vi "FP_Repair_broken_TDMS.vi"(8 "Error in":errorcluster caption="Error In", 11 "TDMS file to repair":path) -> (0 "Error Out":errorcluster caption="Error Out (if any)", 2 "Outcome":string caption="Outcome:")   [LabVIEW 2018]
uses:
  <vilib>/Utility/miscctls.llb/LVPointTypeDef.ctl
  <userlib>/_OpenG.lib/file/file.llb/File Exists - Scalar__ogtk.vi
  <userlib>/_OpenG.lib/file/file.llb/Valid Path - Traditional__ogtk.vi
  <userlib>/_OpenG.lib/file/file.llb/Convert File Extension (Path)__ogtk.vi
panel:
  in  "Repair":bool
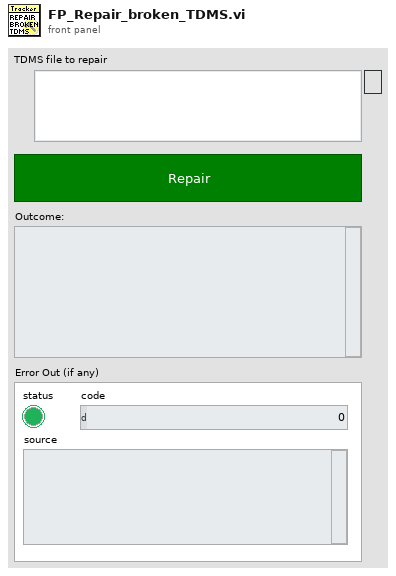
[diagram p1: front panel]
types:
  T1 = enum8{"Enabled", "Disabled", "Disabled and Grayed Out"}
  T2 = typedef "LVPointTypeDef.ctl" = cluster{"Horizontal":i16, "Vertical":i16}
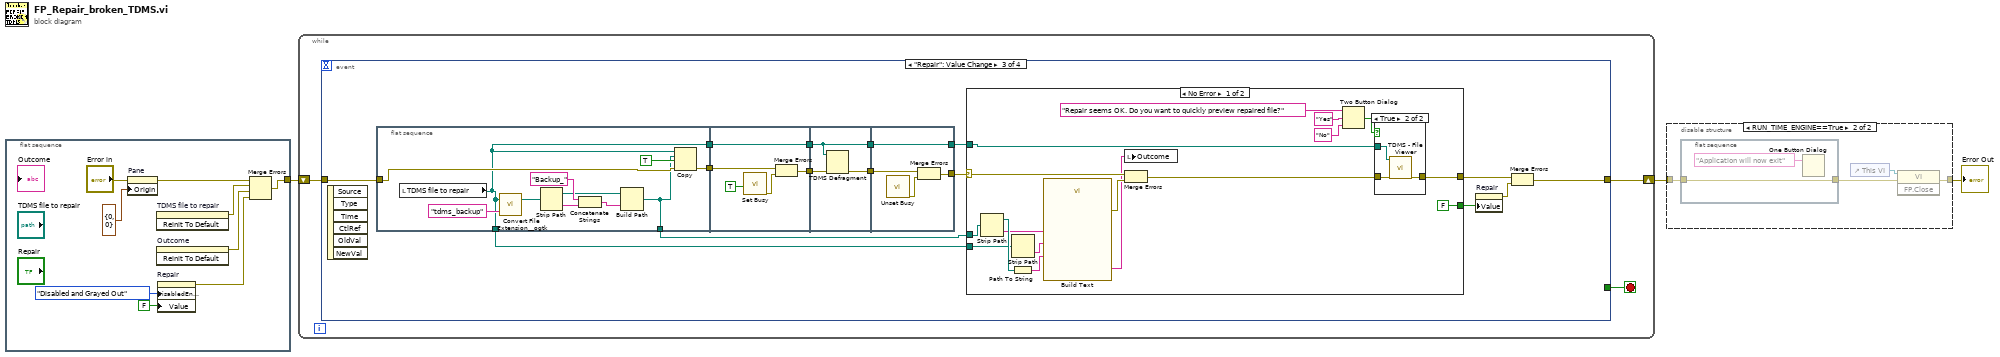
[diagram p0: block diagram]
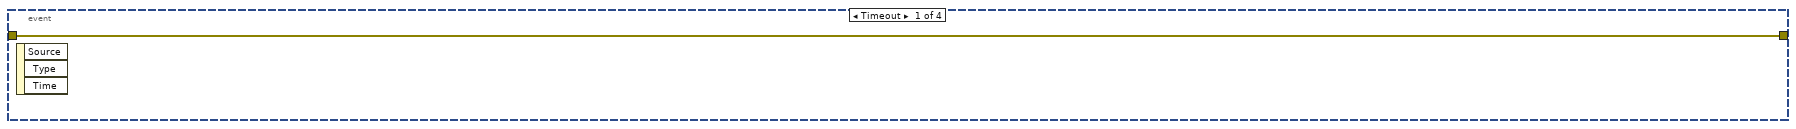
[diagram p3: hidden frame]
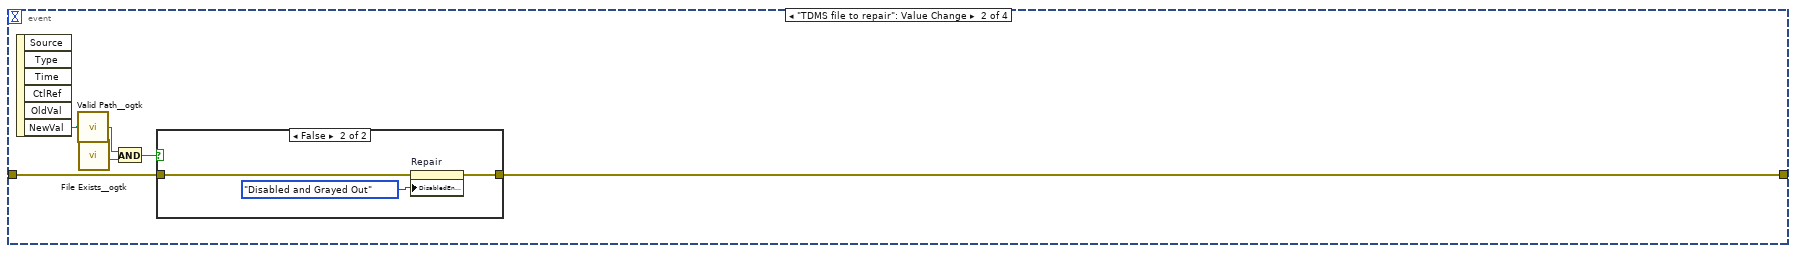
[diagram p4: hidden frame]
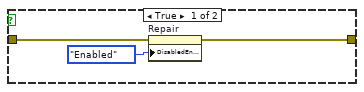
[diagram p5: hidden frame]
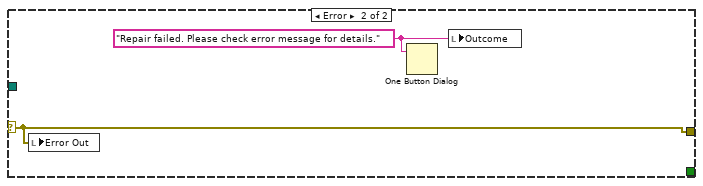
[diagram p7: hidden frame]
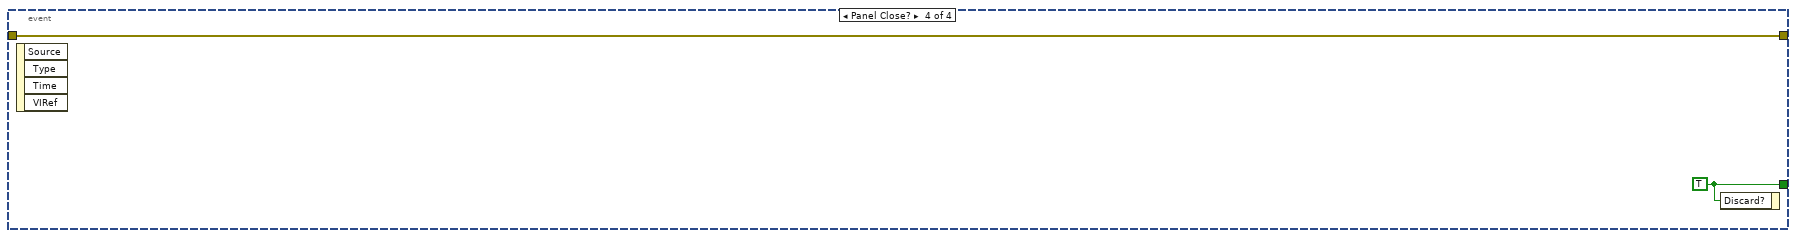
[diagram p8: hidden frame]
diagram:
  n1 = flat-sequence {
    tunnel: [w9] -> w1
    frame #0 {
      n2 = property on="Pane" class="Pane"(error in="Error in", "Origin"=T2 {"Horizontal"=0, "Vertical"=0}) -> (error out=w10:errorcluster)  [unwired: 1 in, 1 out]
      n3 = invoke on="TDMS file to repair" class="Path" method="Reinit To Default"() -> (error out=w6:errorcluster)  [unwired: 3 in, 2 out]
      n4 = invoke on="Outcome" class="Str" method="Reinit To Default"() -> (error out=w5:errorcluster)  [unwired: 3 in, 2 out]
      n5 = property on="Repair" class="Bool (strict)"("DisabledEnum"=T1."Disabled and Grayed Out" ("Disabled"), "Value"=FALSE ("Repair")) -> (error out=w4:errorcluster)  [unwired: 2 in, 1 out]
      n6 = Merge Errors(w10, w6, w5, w4) -> (w9:errorcluster)
    }
  }
  n7 = while {
    shift-right: [w14] -> w3
    shift-left: w1 -> [w13]
    stop <- w15 stop-if-true
    n8 = event shown="[2] \"Repair\": Value Change" {
      selector: _ -> [_ _ _ _]
      dyn-events: _ -> [_ _ _ _]
      timeout: _ -> [_ _ _ _]
      tunnel: [_ _ _ w91] -> w15
      tunnel: [w16 w20 w38 w90] -> w14
      tunnel: w13 -> [w16 w21 w43 w90]
      event Timeout {
        n9 = event-data() -> ()  [unwired: 1 in, 3 out]
      }
      event "TDMS file to repair": Value Change {
        n10 = event-data() -> ("NewVal"=w19:path)  [unwired: 1 in, 5 out]
        n11 = call-poly <userlib>:"Valid Path__ogtk.vi"("path"=w19) -> ("valid"=w22:bool)
        n12 = call-poly <userlib>:"File Exists__ogtk.vi"("file path"=w19) -> ("exists"=w17:bool)  [unwired: 6 in, 1 out]
        n13 = And(x=w22, y=w17) -> (x .and. y?=w18:bool)
        n14 = case shown="False" w18 {
          tunnel: w21 -> [w25 w28]
          tunnel: [w23 w26] -> w20
          frame True {
            n15 = property on="Repair" class="Bool (strict)"(error in=w25, "DisabledEnum"=T1."Enabled" ("Disabled")) -> (error out=w23:errorcluster)  [unwired: 1 in, 1 out]
          }
          frame False {
            n16 = property on="Repair" class="Bool (strict)"(error in=w28, "DisabledEnum"=T1."Disabled and Grayed Out" ("Disabled")) -> (error out=w26:errorcluster)  [unwired: 1 in, 1 out]
          }
        }
      }
      event "Repair": Value Change {
        n17 = event-data() -> ()  [unwired: 1 in, 6 out]
        n18 = flat-sequence {
          tunnel: w43 -> [w75]
          tunnel: [w74] -> w34
          tunnel: [w73] -> w32
          tunnel: [w73] -> w39
          tunnel: [w67] -> w35
          tunnel: w34 -> [w82]
          tunnel: [w79] -> w33
          tunnel: w32 -> [w81]
          tunnel: [w81] -> w31
          tunnel: w33 -> [w85]
          tunnel: w31 -> [w83]
          tunnel: [w84] -> w30
          tunnel: [w83] -> w29
          tunnel: [w88] -> w41
          tunnel: [w87] -> w42
          tunnel: w30 -> [w89]
          tunnel: w29 -> [w88]
          frame #0 {
            n19 = local read "TDMS file to repair"() -> (w73:path)
            n20 = call-poly <userlib>:"Convert File Extension__ogtk.vi"("new ending (none)"="tdms_backup", "file name"=w73) -> ("new filename"=w72:path)  [unwired: 1 out]
            n21 = Strip Path(path=w72) -> (stripped path=w68:path, name=w71:string)
            n22 = Concatenate Strings("Backup_" ("string"), w71) -> (w69:string)
            n23 = Build Path(base path=w68, name or relative path=w69) -> (appended path=w67:path)
            n24 = Copy(8:w75, 9:TRUE ("overwrite (F)"), 10:w67, 11:w73) -> (0:w74:errorcluster)  [unwired: 1 in, 2 out]
          }
          frame #1 {
            n25 = call <vilib>:"Set Busy.vi"("disable click? (T)"=TRUE) -> ("error out"=w78:errorcluster)  [unwired: 9 in, 1 out]
            n26 = Merge Errors(w82, w78) -> (w79:errorcluster)
          }
          frame #2 {
            n27 = TDMS Defragment(4:w85, 7:w83) -> (0:w84:errorcluster)
          }
          frame #3 {
            n28 = call <vilib>:"Unset Busy.vi"() -> ("error out"=w86:errorcluster)  [unwired: 11 in]
            n29 = Merge Errors(w89, w86) -> (w87:errorcluster)
          }
        }
        n30 = case shown="No Error" w42 {
          selector: w42 -> [w56 w66]
          tunnel: w41 -> [w52 _]
          tunnel: [w55 w66] -> w40
          tunnel: w39 -> [w48 _]
          tunnel: [FALSE _] -> w36
          tunnel: w35 -> [w44 _]
          frame No Error {
            n31 = Strip Path(path=w44) -> (stripped path=w51:path, name=w49:string)
            n32 = Path To String(path=w51) -> (string=w50:string)
            n33 = Strip Path(path=w48) -> (name=w47:string)  [unwired: 1 out]
            n34 = call "Build Text"("original_file"=w49, "repaired_file"=w47, "folder"=w50) -> ("Result"=w46:string, "error out"=w53:errorcluster)  [unwired: 11 in]
            n35 = local write "Outcome"(w46) -> ()
            n36 = Merge Errors(w56, w53) -> (w54:errorcluster)
            n37 = Two Button Dialog(message="Repair seems OK. Do you want to quickly preview repaired file?", 1:"No" ("F button name (\"Cancel\")"), 2:"Yes" ("T button name (\"OK\")")) -> (T button?=w59:bool)
            n38 = case shown="True" w59 {
              tunnel: w52 -> [_ w64]
              tunnel: w54 -> [w61 w63]
              tunnel: [w61 w62] -> w55
              frame False {
              }
              frame True {
                n39 = call <vilib>:"TDMS - File Viewer.vi"("error in (no error)"=w63, "file path"=w64) -> ("error out"=w62:errorcluster)  [unwired: 4 in, 1 out]
              }
            }
          }
          frame Error {
            w65 = "Repair failed. Please check error message for details." ("message")
            n40 = local write "Error Out"(w66) -> ()
            n41 = One Button Dialog(message=w65) -> ()  [unwired: 1 in, 1 out]
            n42 = local write "Outcome"(w65) -> ()
          }
        }
        n43 = property on="Repair" class="Bool (strict)"("Value"=w36) -> (error out=w37:errorcluster)  [unwired: 2 in, 1 out]
        n44 = Merge Errors(w40, w37) -> (w38:errorcluster)
      }
      event Panel Close? {
        w91 = TRUE ("Discard?")
        n45 = event-data() -> ()  [unwired: 1 in, 4 out]
        n46 = event-data("Discard?"=w91) -> ()  [unwired: 1 in, 1 out]
      }
    }
  }
  n47 = disable-structure shown="RUN_TIME_ENGINE==True" {
    disable-tunnel: w3 -> [w92 w93]
    disable-tunnel: [w92 w95] -> w2
    frame condition #0 (active) {
    }
    frame condition #1 {
      n48 = flat-sequence {
        tunnel: [w97] -> w94
        tunnel: w93 -> [w97]
        frame #0 {
          n49 = One Button Dialog(message="Application will now exit") -> ()  [unwired: 1 in, 1 out]
        }
      }
      n50 = control-ref of="This VI"() -> (w96:refnum<vi>)
      n51 = invoke class="VI" method="FP.Close"(reference=w96, error in=w94) -> (error out=w95:errorcluster)  [unwired: 1 in, 2 out]
    }
  }
  "Error Out" <- w2
